vi "Shell_NotifyIcon.vi"(4 "error in (no error)":errorcluster, 6 "Operation (NIF_ADD)":T2, 7 "NOTIFYICONDATA":T1) -> (0 "error out":errorcluster)   [LabVIEW 2011]
uses:
  NOTIFYICON_OPERATIONS.ctl
  NOTIFYICONDATA.ctl
  SHELL32.DLL
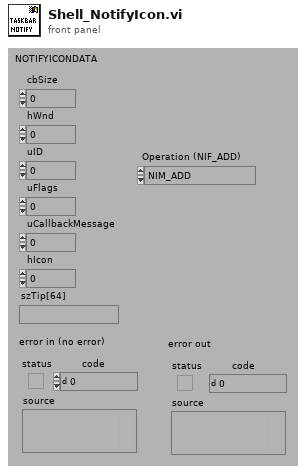
[diagram p1: front panel]
types:
  T1 = typedef "NOTIFYICONDATA.ctl" = cluster{"cbSize":i32, "hWnd":i32, "uID":i32, "uFlags":i32, "uCallbackMessage":i32, "hIcon":i32, "szTip[64]":string}
  T2 = typedef "NOTIFYICON_OPERATIONS.ctl" = enum16{"NIM_ADD", "NIM_MODIFY", "NIM_DELETE", "NIM_SETFOCUS", "NIM_SETVERSION"}
  T3 = cluster{"cbSize":i32, "hWnd":i32, "uID":i32, "uFlags":i32, "uCallbackMessage":i32, "hIcon":i32}
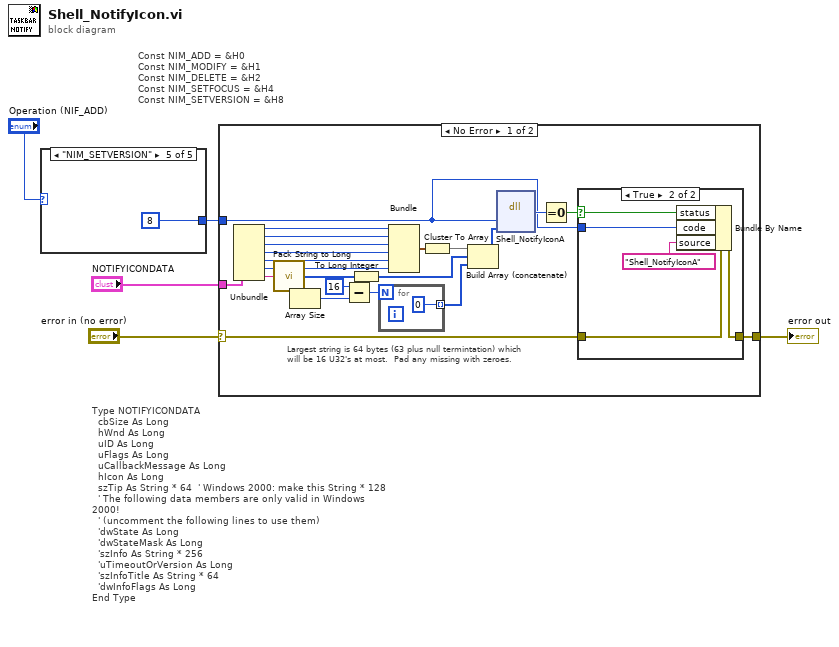
[diagram p0: block diagram]
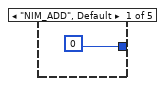
[diagram p2: hidden frame]
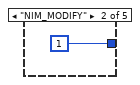
[diagram p3: hidden frame]
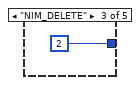
[diagram p4: hidden frame]
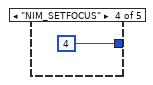
[diagram p5: hidden frame]
diagram:
  # "Type NOTIFYICONDATA\n  cbSize As Long\n  hWnd As Long\n  uID As Long\n  uFlags As Long\n  uCallbackMessage As Long\n  hIcon As Long\n  szTip As String * 64  ' Windows 2000: make this String * 128\n  ' The following data members are only valid in Windows 2000!\n  ' (uncomment the following lines to use them)\n  'dwState As Long\n  'dwStateMask As Long\n  'szInfo As String * 256\n  'uTimeoutOrVersion As Long\n  'szInfoTitle As String * 64\n  'dwInfoFlags As Long\nEnd Type"
  # "Const NIM_ADD = &H0\nConst NIM_MODIFY = &H1\nConst NIM_DELETE = &H2\nConst NIM_SETFOCUS = &H4\nConst NIM_SETVERSION = &H8"
  n1 = case shown="\"NIM_SETVERSION\"" "Operation (NIF_ADD)" {
    tunnel: [0 1 2 4 8] -> w1
    frame "NIM_ADD", Default {
    }
    frame "NIM_MODIFY" {
    }
    frame "NIM_DELETE" {
    }
    frame "NIM_SETFOCUS" {
    }
    frame "NIM_SETVERSION" {
    }
  }
  n2 = case shown="No Error" "error in (no error)" {
    selector: "error in (no error)" -> [w30 w40]
    tunnel: "NOTIFYICONDATA" -> [w28 _]
    tunnel: [w29 w40] -> w4
    tunnel: w1 -> [w22 _]
    frame No Error {
      # "Largest string is 64 bytes (63 plus null termintation) which\nwill be 16 U32's at most.  Pad any missing with zeroes."
      n3 = Unbundle(w28) -> ("cbSize"=w12:i32, "hWnd"=w27:i32, "uID"=w13:i32, "uFlags"=w26:i32, "uCallbackMessage"=w25:i32, "hIcon"=w24:i32, "szTip[64]"=w19:string)
      n4 = call "Pack String to Long.vi"("string"=w19) -> ("packed"=w18:u32[])  [unwired: 4 out]
      n5 = Array Size(array=w18) -> (size(s)=w16:i32)
      n6 = Subtract(x=16, y=w16) -> (x-y=w15:i32)
      n7 = To Long Integer(number=w18) -> (32bit integer=w11:i32[])
      n8 = for {
        N: w15 -> [_]
        tunnel: [0] -> w14 mode=indexing
      }
      n9 = Bundle("cbSize"=w12, "hWnd"=w27, "uID"=w13, "uFlags"=w26, "uCallbackMessage"=w25, "hIcon"=w24) -> (w23:T3)  [unwired: 1 out]
      n10 = Cluster To Array(cluster=w23) -> (array=w21:i32[])
      n11 = Build Array (concatenate)(w21, w11, w14) -> (w20:i32[])
      n12 = dll-call lib="SHELL32.DLL" fn="Shell_NotifyIconA"("dwMessage"=w22, "pnid"=w20) -> (w32:i32)  [unwired: 5 in, 2 out]
      n13 = Equal To 0?(x=w32) -> (x = 0?=w31:bool)
      n14 = case shown="True" w31 {
        selector: w31 -> [_ w38]
        tunnel: w30 -> [w34 w39]
        tunnel: [w34 w37] -> w29
        tunnel: w22 -> [_ w35]
        frame False {
        }
        frame True {
          n15 = Bundle By Name(cluster=w39, "status"=w38, "code"=w35, "source"="Shell_NotifyIconA") -> (w37:errorcluster)
        }
      }
    }
    frame Error {
    }
  }
  "error out" <- w4
